vi "DriveBegin.vi"(8 "error in (no error)":errorcluster) -> (0 "error out":errorcluster)   [LabVIEW 2020]
doc: "Begin for Drive\n\nInputs:\n -- Error in -- Error cluster -- propagated error input\n\nOutputs:\n -- Error out -- Error cluster -- progated error output"
uses:
  <vilib>/Rock Robotics/SystemInterfaces/DIO/FPGA_DIOPWMChannel.ctl
  <vilib>/Rock Robotics/WPI/Encoder/WPI_EncoderType.ctl
  <vilib>/Rock Robotics/SystemInterfaces/DIO/FPGA_DIOChannel.ctl
  <vilib>/Rock Robotics/WPI/ThirdParty/Phoenix-LabVIEW/Motor Controller/Controls/CTRE_Phoenix_MotorControl_NeutralMode.ctl
  DriveGlobal.vi
  <vilib>/Rock Robotics/WPI/Counter/WPI_CounterDigitalInputToDigitalSource.vi
  <vilib>/Rock Robotics/WPI/ThirdParty/JAS_Junk/TrajLib/Trajectory_Library.lvlib
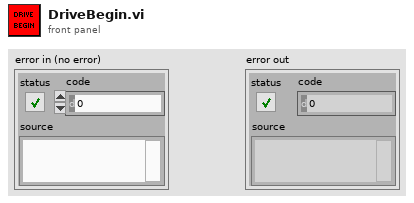
[diagram p1: front panel]
types:
  T1 = typedef "FPGA_DIOPWMChannel.ctl" = enum8{"PWM 0", "PWM 1", "PWM 2", "PWM 3", "PWM 4", "PWM 5", "PWM 6", "PWM 7", "PWM 8", "PWM 9", "PWM MXP 0", "PWM MXP 1", "PWM MXP 2", "PWM MXP 3", "PWM MXP 4", "PWM MXP 5", "PWM MXP 6", "PWM MXP 7", "PWM MXP 8", "PWM MXP 9", "Invalid"}
  T2 = typedef "WPI_EncoderType.ctl" = enum16{"1x", "2x", "4x"}
  T3 = typedef "FPGA_DIOChannel.ctl" = enum8{"DIO 0", "DIO 1", "DIO 2", "DIO 3", "DIO 4", "DIO 5", "DIO 6", "DIO 7", "DIO 8", "DIO 9", "DIO MXP 0", "DIO MXP 1", "DIO MXP 2", "DIO MXP 3", "DIO MXP 4", "DIO MXP 5", "DIO MXP 6", "DIO MXP 7", "DIO MXP 8", "DIO MXP 9", "DIO MXP 10", "DIO MXP 11", "DIO MXP 12", "DIO MXP 13", "DIO MXP 14", "DIO MXP 15", "SPI Port CS1", "SPI Port CS2", "SPI Port CS3", "SPI Port MISO", "SPI Port MOSI", "Invalid"}
  T4 = typedef "CTRE_Phoenix_MotorControl_NeutralMode.ctl" = enum8{"EEPROMSetting", "Override to Coast", "Override to Brake"}
  T5 = typedef "Trajectory_Library.lvlib/TRANSLATION2D.ctl" = cluster{"X":dbl, "Y":dbl}
  T6 = typedef "WPI_MotorControlDeviceRef.ctl" = cluster{"DeviceStatus":errorcluster, "Type":T7, "PWM":cluster{"PWM Channel":T1, "DeadBand":T8}, "CAN":cluster{"Device Number":u8, "SetOutput VI Ref":variant, "GetOutput VI Ref":variant, "Enable VI Ref":variant, "Disable VI Ref":variant, "Data":variant}, "Invert":bool, "DIO PWM":cluster{"PWM \"Enable\" Channel":T1, "DIOChannel":T3, "PWM Rate":dbl}}
  T7 = typedef "WPI_MotorControlType.ctl" = enum16{"PWM", "CAN", "DIO PWM"}
  T8 = typedef "WPI_PWMDeadband.ctl" = cluster{"Name":string, "maxPositivePwm":i32, "minPositivePwm":i32, "centerPwm":i32, "maxNegativePwm":i32, "minNegativePwm":i32, "angularRange":u16}
  T9 = typedef "Trajectory_Library.lvlib/SWERVE_DRIVE_KINEMATICS.ctl" = cluster{"NumModules":i32, "InverseKinematics":T10, "ForwardKinematics":T10, "Modules":T5[], "PrevCoR":T5, "SavedModuleStates":T11[]}
  T10 = typedef "NI_Matrix.lvlib/RealMatrix.ctl" = dbl[][]
  T11 = typedef "Trajectory_Library.lvlib/SWERVE_DRIVE_MODULE_STATE.ctl" = cluster{"Speed":dbl, "Angle":T12}
  T12 = typedef "Trajectory_Library.lvlib/ROTATION2D.ctl" = cluster{"VALUE":dbl, "COS":dbl, "SIN":dbl}
  T13 = typedef "WPI_DigitalInputDevRef.ctl" = cluster{"DevStatus":errorcluster, "DIO Channel":T3}
  T14 = typedef "FPGA_CounterEncoderSourceConvertionLVSourceType.ctl" = cluster{"DevStatus":errorcluster, "AnalogTriggerMode?":bool, "DigitalMode":cluster{"DIO Channel":T15}, "AnalogTriggerMode":cluster{"AnalogTriggerIndex":T16, "OutputType":T17}}
  T15 = typedef "FPGA_DIODigitalSourceChannel.ctl" = enum8{"DIO 0", "DIO 1", "DIO 2", "DIO 3", "DIO 4", "DIO 5", "DIO 6", "DIO 7", "DIO 8", "DIO 9", "DIO MXP 0", "DIO MXP 1", "DIO MXP 2", "DIO MXP 3", "DIO MXP 4", "DIO MXP 5", "DIO MXP 6", "DIO MXP 7", "DIO MXP 8", "DIO MXP 9", "DIO MXP 10", "DIO MXP 11", "DIO MXP 12", "DIO MXP 13", "DIO MXP 14", "DIO MXP 15", "SPI Port CS1", "SPI Port CS2", "SPI Port CS3", "SPI Port MISO", "SPI Port MOSI", "Disabled"}
  T16 = typedef "FPGA_AnalogTriggerIndex.ctl" = enum8{"Trig 0", "Trig 1", "Trig 2", "Trig 3", "Trig 4", "Trig 5", "Trig 6", "Trig 7", "Invalid"}
  T17 = typedef "FPGA_AnalogTriggerOutType.ctl" = enum16{"InWindow", "TriggerState", "Rising", "Falling"}
  T18 = typedef "WPI_EncoderDevRef.ctl" = cluster{"DevStatus":errorcluster, "EncoderIndex":T19, "CounterIndex":T20, "DistancePerCount":dbl, "Decoding Type":T2}
  T19 = typedef "FPGA_EncoderIdx.ctl" = enum8{"Enc 0", "Enc 1", "Enc 2", "Enc 3", "Enc 4", "Enc 5", "Enc 6", "Enc 7", "Invalid"}
  T20 = typedef "FPGA_CounterCtrSystemIndex.ctl" = enum8{"Ctr 0", "Ctr 1", "Ctr 2", "Ctr 3", "Ctr 4", "Ctr 5", "Ctr 6", "Ctr 7", "Invalid"}
  T21 = typedef "WPI_PWMDeviceRef.ctl" = cluster{"DeviceStatus":errorcluster, "PWM Channel":T1}
  T22 = typedef "ADIS16470 Device Reference.ctl" = cluster{"DevStatus":errorcluster, "Hardware Config":T23, "Calibration Complete":refnum<notifier>, "Status Reference":refnum<data-value>, "Data Reference":refnum<data-value>, "Sychronous Process VI":T26, "Cmd FIFO":refnum<k33>, "Source":T14, "Data FIFO":refnum<k33>, "Calibration Time (ms)":u32, "Data Reference":refnum<data-value>}
  T23 = typedef "ADIS16470 Hardware Configuration.ctl" = cluster{"SPI Clock Rate (Hz)":dbl, "IMU SPI Mode (3)":T24, "IMU Reset Pin":T3, "IMU SPI Bus":T25, "IMU Data Ready Pin":T3, "Stall Config":cluster{"Pow2BytesPerRead":u8, "StallTicks":u16, "CsToSclkTicks":u8}}
  T24 = typedef "WPI_SPIMode.ctl" = enum16{"Mode 0 (Clk Idle Low,Sample on Leading)", "Mode 1 (Clk Idle Low,Sample on Trailing)", "Mode 2 (Clk Idle High,Sample on Leading)", "Mode 3 (Clk Idle High,Sample on Trailing)"}
  T25 = typedef "spi_bus.ctl" = enum16{"SPI On-Board, CS0", "SPI On-Board, CS1", "SPI On-Board, CS2", "SPI On-Board, CS3", "SPI MXP", "Invalid"}
  T26 = typedef "ADIS16470 Process.ctl" = refnum<vi>
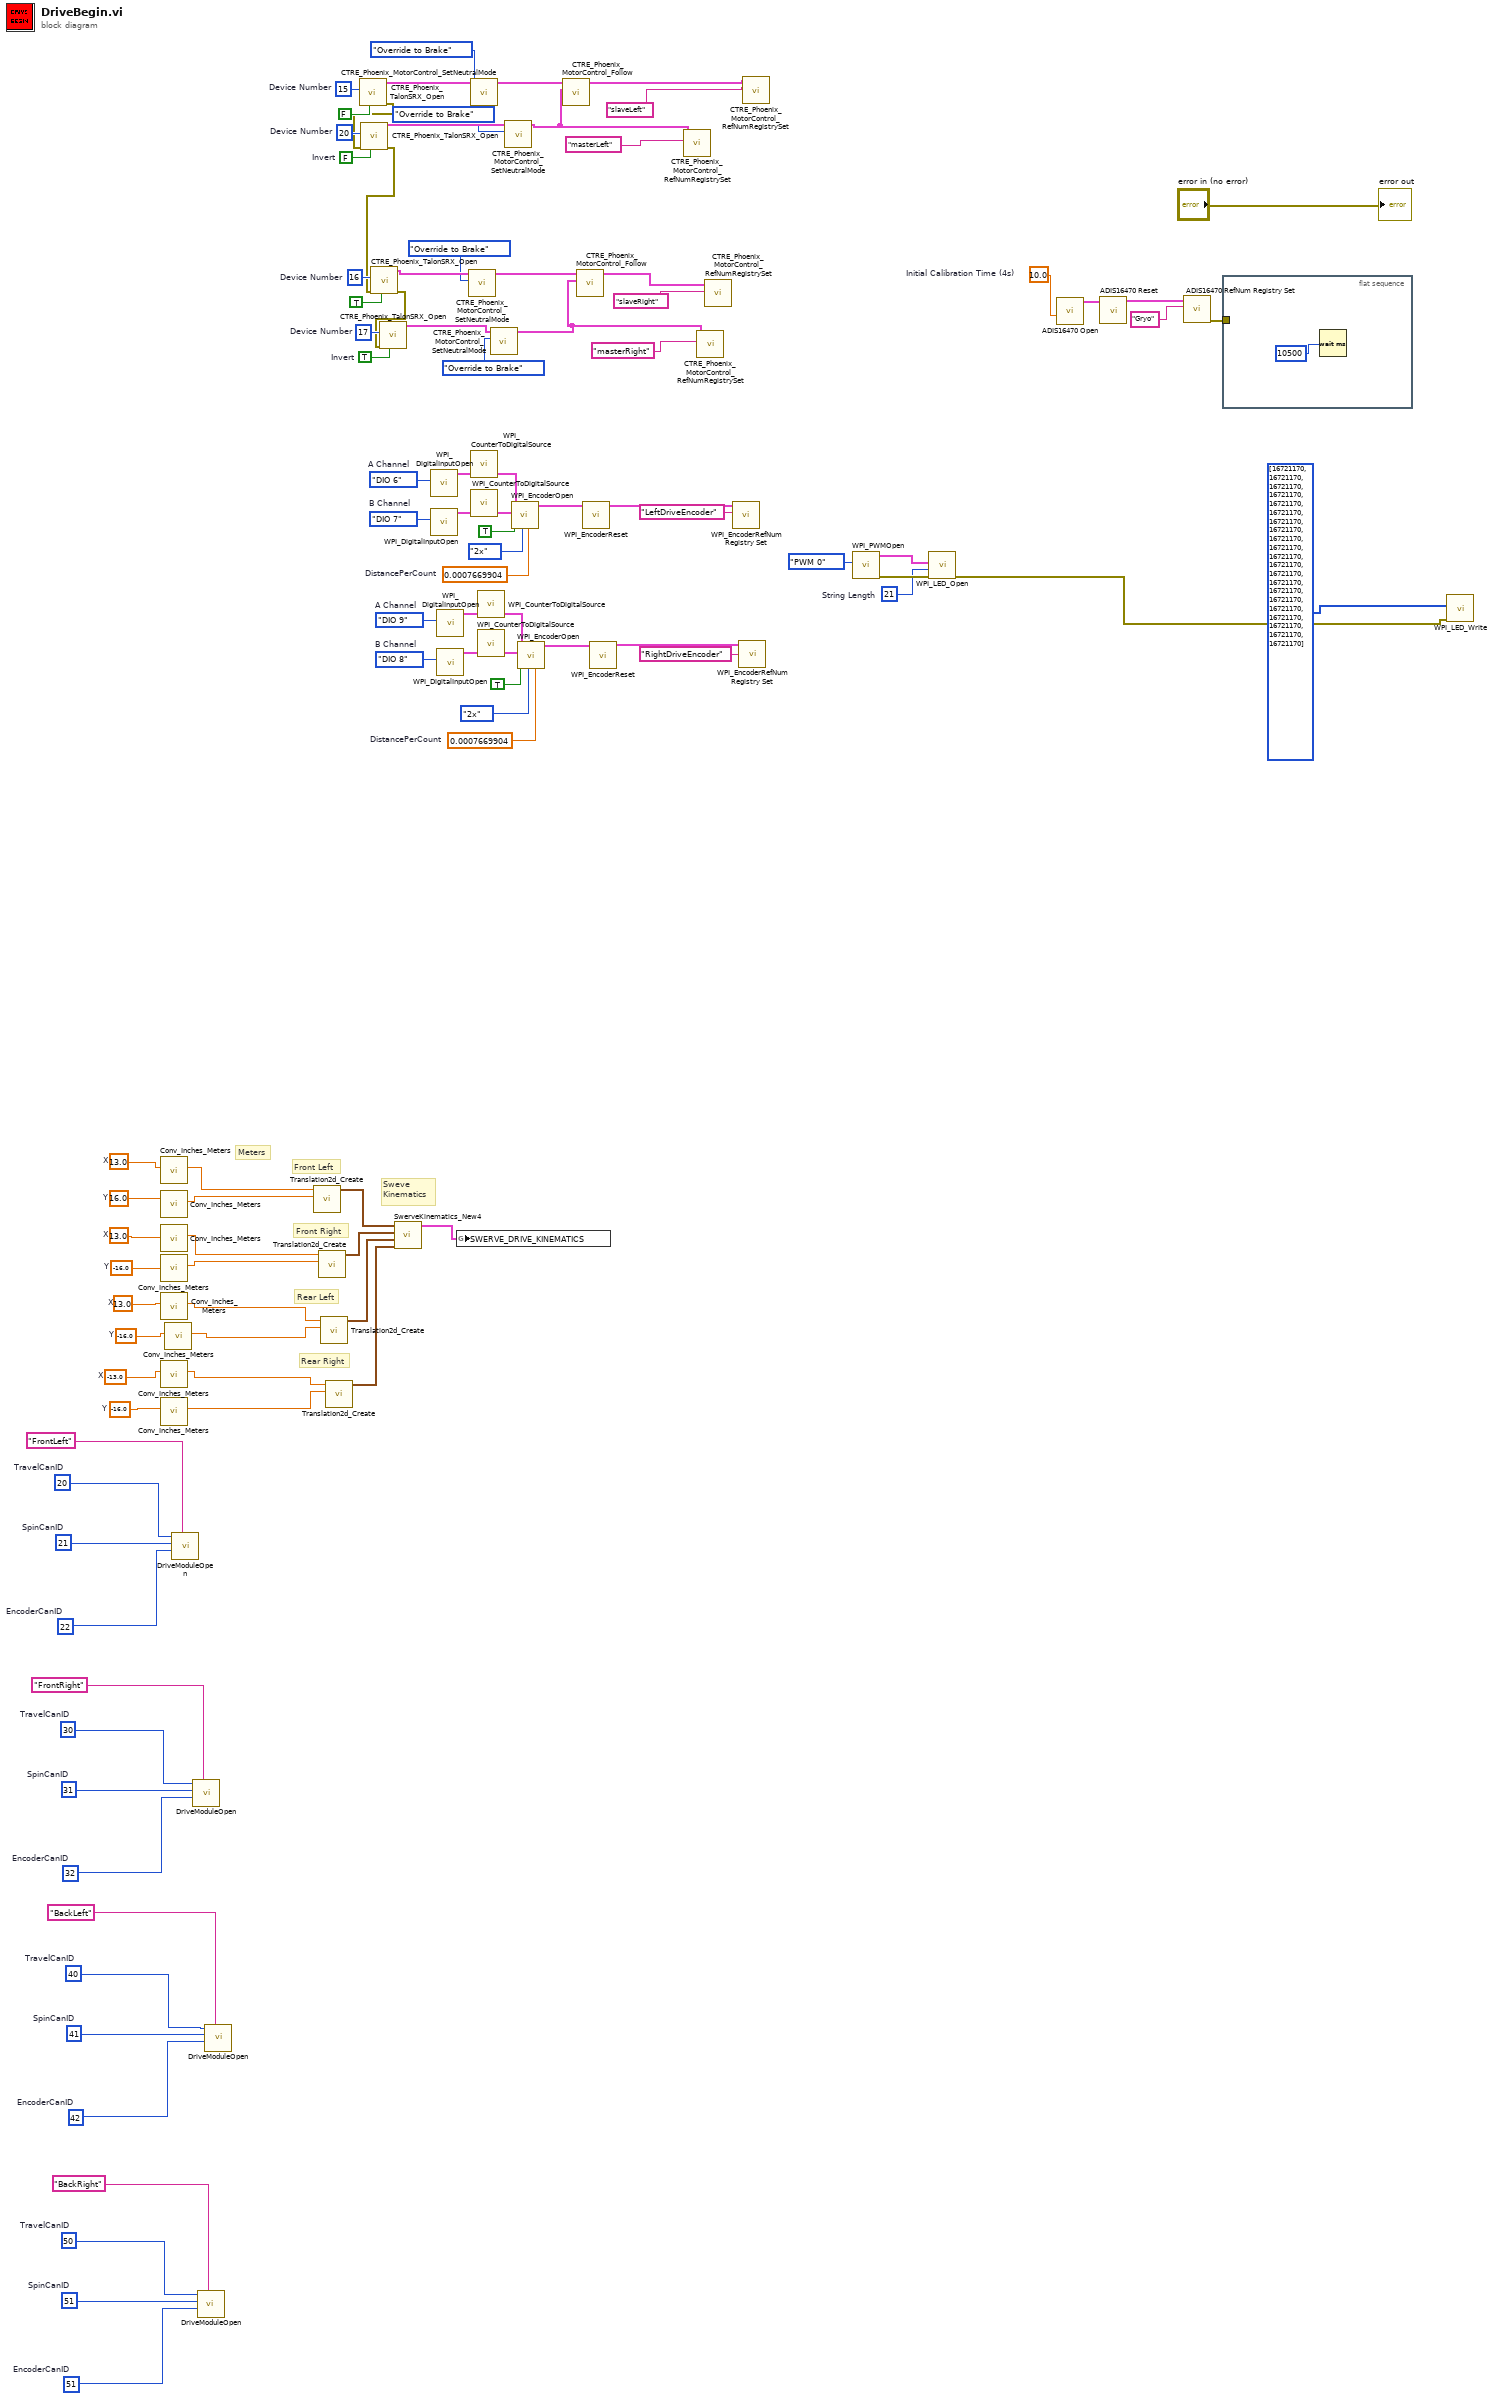
[diagram p0: block diagram]
diagram:
  w3 = u8 50  # TravelCanID
  w2 = u8 51  # SpinCanID
  w1 = u8 51  # EncoderCanID
  w6 = u8 40  # TravelCanID
  w5 = u8 41  # SpinCanID
  w4 = u8 42  # EncoderCanID
  w9 = u8 30  # TravelCanID
  w8 = u8 31  # SpinCanID
  w7 = u8 32  # EncoderCanID
  w10 = u8 20  # TravelCanID
  w11 = u8 21  # SpinCanID
  w12 = u8 22  # EncoderCanID
  w19 = -13.0  # X
  w18 = -16.0  # Y
  w21 = 13.0  # X
  w20 = -16.0  # Y
  w23 = 13.0  # X
  w22 = -16.0  # Y
  w25 = 13.0  # X
  w24 = 16.0  # Y
  w41 = u16 21  # String Length
  w45 = 0.0007669904  # DistancePerCount
  w47 = 0.0007669904  # DistancePerCount
  w59 = FPGA_DIOChannel."DIO 8"  # B Channel
  w58 = FPGA_DIOChannel."DIO 9"  # A Channel
  w65 = FPGA_DIOChannel."DIO 7"  # B Channel
  w64 = FPGA_DIOChannel."DIO 6"  # A Channel
  w74 = u8 16  # Device Number
  w75 = u8 15  # Device Number
  w94 = 10.0  # Initial Calibration Time (4s)
  w96 = FALSE  # Invert
  w97 = TRUE  # Invert
  w99 = u8 17  # Device Number
  w98 = u8 20  # Device Number
  # "Meters"
  # "Sweve\nKinematics"
  # "Rear Right"
  # "Rear Left"
  # "Front Right"
  # "Front Left"
  n1 = call <vilib>:"Conv_Inches_Meters.vi"("INCH"=w25) -> ("Meters"=w26:dbl)  [unwired: 10 in]
  n2 = call <vilib>:"Conv_Inches_Meters.vi"("INCH"=w24) -> ("Meters"=w27:dbl)  [unwired: 10 in]
  n3 = call <vilib>:"Conv_Inches_Meters.vi"("INCH"=w23) -> ("Meters"=w28:dbl)  [unwired: 10 in]
  n4 = call <vilib>:"Conv_Inches_Meters.vi"("INCH"=w22) -> ("Meters"=w29:dbl)  [unwired: 10 in]
  n5 = call <vilib>:"Conv_Inches_Meters.vi"("INCH"=w21) -> ("Meters"=w30:dbl)  [unwired: 10 in]
  n6 = call <vilib>:"Conv_Inches_Meters.vi"("INCH"=w19) -> ("Meters"=w33:dbl)  [unwired: 10 in]
  n7 = call <vilib>:"Conv_Inches_Meters.vi"("INCH"=w18) -> ("Meters"=w32:dbl)  [unwired: 10 in]
  n8 = call <vilib>:"Conv_Inches_Meters.vi"("INCH"=w20) -> ("Meters"=w31:dbl)  [unwired: 10 in]
  n9 = call "DriveModuleOpen.vi"("ModualNamePrefix"="FrontLeft", "EncoderCanID"=w12, "SpinCanID"=w11, "TravelCanID"=w10) -> ()  [unwired: 7 in, 1 out]
  n10 = call "DriveModuleOpen.vi"("ModualNamePrefix"="FrontRight", "EncoderCanID"=w7, "SpinCanID"=w8, "TravelCanID"=w9) -> ()  [unwired: 7 in, 1 out]
  n11 = call "DriveModuleOpen.vi"("ModualNamePrefix"="BackRight", "EncoderCanID"=w1, "SpinCanID"=w2, "TravelCanID"=w3) -> ()  [unwired: 7 in, 1 out]
  n12 = call "DriveModuleOpen.vi"("ModualNamePrefix"="BackLeft", "EncoderCanID"=w4, "SpinCanID"=w5, "TravelCanID"=w6) -> ()  [unwired: 7 in, 1 out]
  n13 = call <vilib>:"Translation2d_Create.vi"("Y"=w27, "X"=w26) -> ("TRANSLATION"=w34:T5)  [unwired: 9 in]
  n14 = call <vilib>:"Translation2d_Create.vi"("Y"=w29, "X"=w28) -> ("TRANSLATION"=w35:T5)  [unwired: 9 in]
  n15 = call <vilib>:"Translation2d_Create.vi"("Y"=w31, "X"=w30) -> ("TRANSLATION"=w36:T5)  [unwired: 9 in]
  n16 = call <vilib>:"Translation2d_Create.vi"("Y"=w32, "X"=w33) -> ("TRANSLATION"=w37:T5)  [unwired: 9 in]
  n17 = call <vilib>:"CTRE_Phoenix_TalonSRX_Open.vi"("Invert"=FALSE, "Device Number"=w75) -> ("error out"=w70:errorcluster, "PhoenixMotorControlDevRef"=w86:T6)  [unwired: 8 in]
  n18 = call <vilib>:"CTRE_Phoenix_TalonSRX_Open.vi"("Invert"=w96, "error in"=w70, "Device Number"=w98) -> ("error out"=w69:errorcluster, "PhoenixMotorControlDevRef"=w89:T6)  [unwired: 7 in]
  n19 = call <vilib>:"CTRE_Phoenix_TalonSRX_Open.vi"("Invert"=TRUE, "error in"=w69, "Device Number"=w74) -> ("error out"=w68:errorcluster, "PhoenixMotorControlDevRef"=w80:T6)  [unwired: 7 in]
  n20 = call <vilib>:"CTRE_Phoenix_TalonSRX_Open.vi"("Invert"=w97, "error in"=w68, "Device Number"=w99) -> ("PhoenixMotorControlDevRef"=w91:T6)  [unwired: 7 in, 1 out]
  n21 = call <vilib>:"SwerveKinematics_New4.vi"("wheel 3"=w37, "wheel 2"=w36, "wheel 1"=w35, "wheel 0"=w34) -> ("SWERVE_DRIVE_KINEMATICS"=w17:T9)  [unwired: 7 in]
  n22 = call <vilib>:"WPI_DigitalInputOpen.vi"("DIO Channel"=w64) -> ("DigitalInputDevRef"=w62:T13)  [unwired: 1 in, 9 out]
  n23 = call <vilib>:"WPI_DigitalInputOpen.vi"("DIO Channel"=w65) -> ("DigitalInputDevRef"=w63:T13)  [unwired: 1 in, 9 out]
  n24 = call <vilib>:"WPI_DigitalInputOpen.vi"("DIO Channel"=w58) -> ("DigitalInputDevRef"=w56:T13)  [unwired: 1 in, 9 out]
  n25 = call <vilib>:"WPI_DigitalInputOpen.vi"("DIO Channel"=w59) -> ("DigitalInputDevRef"=w57:T13)  [unwired: 1 in, 9 out]
  n26 = global write "DriveGlobal.vi" "SWERVE_DRIVE_KINEMATICS"(w17) -> ()
  n27 = call <vilib>:"CTRE_Phoenix_MotorControl_SetNeutralMode.vi"("Motor Control Neutral Mode"=CTRE_Phoenix_MotorControl_NeutralMode."Override to Brake", "PhoenixMotorControlDevRef"=w80) -> ("PhoenixMotorControlDevRef"=w79:T6)  [unwired: 8 in, 1 out]
  n28 = call <vilib>:"CTRE_Phoenix_MotorControl_SetNeutralMode.vi"("Motor Control Neutral Mode"=CTRE_Phoenix_MotorControl_NeutralMode."Override to Brake", "PhoenixMotorControlDevRef"=w86) -> ("PhoenixMotorControlDevRef"=w84:T6)  [unwired: 8 in, 1 out]
  n29 = call-poly <vilib>:"WPI_CounterToDigitalSource.vi"("DigitalInputDevRef"=w62) -> ("Digital Source"=w66:T14)  [unwired: 6 out]
  n30 = call-poly <vilib>:"WPI_CounterToDigitalSource.vi"("DigitalInputDevRef"=w63) -> ("Digital Source"=w67:T14)  [unwired: 6 out]
  n31 = call-poly <vilib>:"WPI_CounterToDigitalSource.vi"("DigitalInputDevRef"=w56) -> ("Digital Source"=w60:T14)  [unwired: 6 out]
  n32 = call-poly <vilib>:"WPI_CounterToDigitalSource.vi"("DigitalInputDevRef"=w57) -> ("Digital Source"=w61:T14)  [unwired: 6 out]
  n33 = call <vilib>:"CTRE_Phoenix_MotorControl_SetNeutralMode.vi"("Motor Control Neutral Mode"=CTRE_Phoenix_MotorControl_NeutralMode."Override to Brake", "PhoenixMotorControlDevRef"=w91) -> ("PhoenixMotorControlDevRef"=w71:T6)  [unwired: 8 in, 1 out]
  n34 = call <vilib>:"CTRE_Phoenix_MotorControl_SetNeutralMode.vi"("Motor Control Neutral Mode"=CTRE_Phoenix_MotorControl_NeutralMode."Override to Brake", "PhoenixMotorControlDevRef"=w89) -> ("PhoenixMotorControlDevRef"=w83:T6)  [unwired: 8 in, 1 out]
  n35 = call <vilib>:"WPI_EncoderOpen.vi"("DistancePerCount"=w47, "Decoding Type"=WPI_EncoderType."2x", "Invert Direction (False)"=TRUE, "BSource"=w67, "ASource"=w66) -> ("EncoderDevRef"=w53:T18)  [unwired: 5 in, 1 out]
  n36 = call <vilib>:"WPI_EncoderOpen.vi"("DistancePerCount"=w45, "Decoding Type"=WPI_EncoderType."2x", "Invert Direction (False)"=TRUE, "BSource"=w61, "ASource"=w60) -> ("EncoderDevRef"=w55:T18)  [unwired: 5 in, 1 out]
  n37 = call <vilib>:"CTRE_Phoenix_MotorControl_Follow.vi"("Master Controller to Follow"=w83, "PhoenixMotorControlDevRef"=w84) -> ("PhoenixMotorControlDevRef"=w82:T6)  [unwired: 8 in, 1 out]
  n38 = call <vilib>:"CTRE_Phoenix_MotorControl_Follow.vi"("Master Controller to Follow"=w71, "PhoenixMotorControlDevRef"=w79) -> ("PhoenixMotorControlDevRef"=w78:T6)  [unwired: 8 in, 1 out]
  n39 = call <vilib>:"WPI_EncoderReset.vi"("EncoderDevRef"=w53) -> ("EncoderDevRef"=w52:T18)  [unwired: 9 in, 1 out]
  n40 = call <vilib>:"WPI_EncoderReset.vi"("EncoderDevRef"=w55) -> ("EncoderDevRef"=w54:T18)  [unwired: 9 in, 1 out]
  n41 = call <vilib>:"CTRE_Phoenix_MotorControl_RefNumRegistrySet.vi"("refnum name"="masterLeft", "PhoenixMotorControlDevRef"=w83) -> ()  [unwired: 8 in, 2 out]
  n42 = call <vilib>:"CTRE_Phoenix_MotorControl_RefNumRegistrySet.vi"("refnum name"="masterRight", "PhoenixMotorControlDevRef"=w71) -> ()  [unwired: 8 in, 2 out]
  n43 = call <vilib>:"CTRE_Phoenix_MotorControl_RefNumRegistrySet.vi"("refnum name"="slaveRight", "PhoenixMotorControlDevRef"=w78) -> ()  [unwired: 8 in, 2 out]
  n44 = call <vilib>:"WPI_EncoderRefNum Registry Set.vi"("refnum name"="LeftDriveEncoder", "EncoderDevRef"=w52) -> ()  [unwired: 8 in, 2 out]
  n45 = call <vilib>:"WPI_EncoderRefNum Registry Set.vi"("refnum name"="RightDriveEncoder", "EncoderDevRef"=w54) -> ()  [unwired: 8 in, 2 out]
  n46 = call <vilib>:"CTRE_Phoenix_MotorControl_RefNumRegistrySet.vi"("refnum name"="slaveLeft", "PhoenixMotorControlDevRef"=w82) -> ()  [unwired: 8 in, 2 out]
  n47 = call <vilib>:"WPI_PWMOpen.vi"("PWM Channel"=FPGA_DIOPWMChannel."PWM 0") -> ("error out"=w42:errorcluster, "PWMDeviceRef"=w43:T21)  [unwired: 9 in]
  n48 = call <vilib>:"WPI_LED_Open.vi"("error in"=w42, "String Length"=w41, "PWMDeviceRef"=w43) -> ("error out"=w38:errorcluster)  [unwired: 8 in]
  n49 = call <vilib>:"ADIS16470 Open.vi"("Initial Calibration Time (4s)"=w94) -> ("ADIS16470DevRef"=w93:T22)  [unwired: 9 in, 1 out]
  n50 = call <vilib>:"ADIS16470 Reset.vi"("ADIS16470DevRef"=w93) -> ("ADIS16470DevRef"=w92:T22)  [unwired: 9 in, 1 out]
  n51 = call <vilib>:"ADIS16470 RefNum Registry Set.vi"("refnum name"="Gryo", "ADIS16470DevRef in"=w92) -> ("error out"=w87:errorcluster)  [unwired: 8 in, 1 out]
  n52 = flat-sequence {
    tunnel: w87 -> [_]
    frame #0 {
      n53 = Wait (ms)(milliseconds to wait=u32 10500) -> ()  [unwired: 1 out]
    }
  }
  n54 = call <vilib>:"WPI_LED_Write.vi"("error in"=w38, "Color Array"=u32[] [16721170, 16721170, 16721170, 16721170, 16721170, 16721170, 16721170, 16721170, 16721170, 16721170, 16721170, 16721170, 16721170, 16721170, 16721170, 16721170, 16721170, 16721170, 16721170, 16721170, 16721170]) -> ()  [unwired: 9 in, 1 out]
  "error out" <- "error in (no error)"
